vi "ReadMNValuesJSON_EditTolerance.vi"(7 "Default JSON\nVariant in":variant, 8 "error in":errorcluster, 9 "Part Name":string, 10 "Rack Number":string, 11 "JSON file path":path=path "C:/Users/raakeshs/Desktop/ppts/JSON/Write to JSON String/data/Files/test4.json") -> (0 "error out":errorcluster, 3 "Rack Controller Parameters":T1)   [LabVIEW 2015, in "ZenGage v3.0 UI.lvclass"]
uses:
  ZenGage v3.0 UI.lvclass
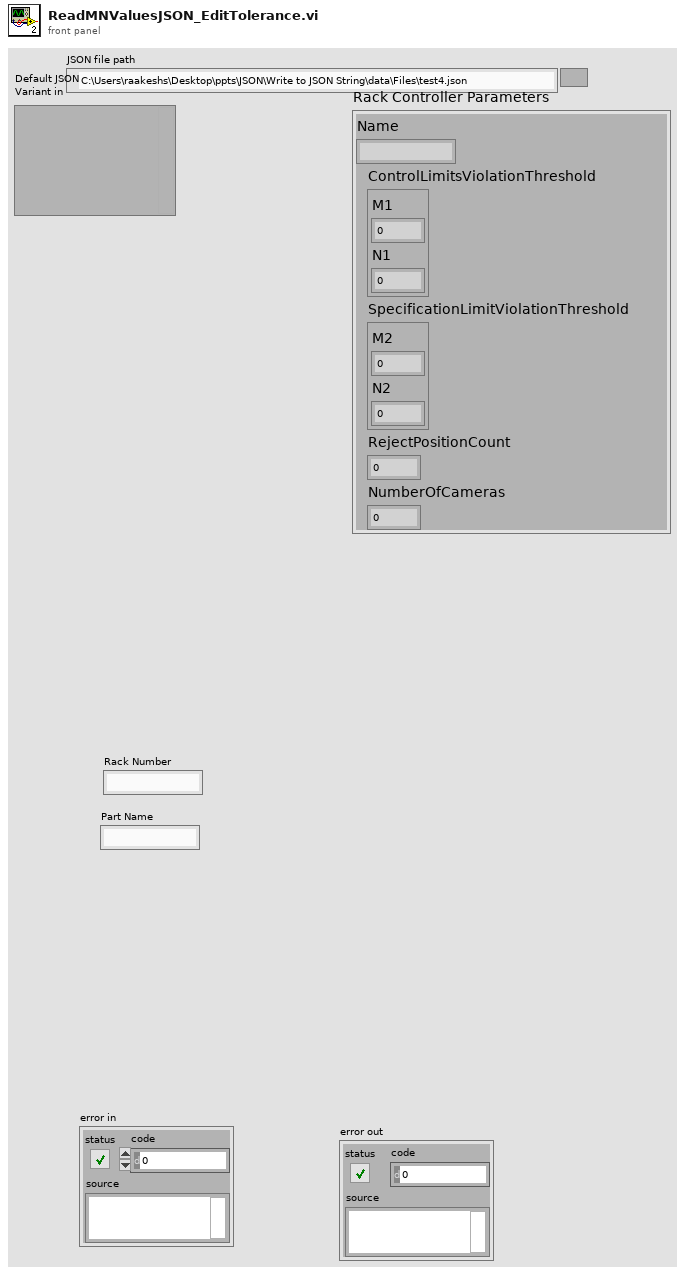
[diagram p1: front panel]
types:
  T1 = cluster{"Name":string, "ControlLimitsViolationThreshold":cluster{"M1":i32, "N1":i32}, "SpecificationLimitViolationThreshold":cluster{"M2":i32, "N2":i32}, "RejectPositionCount":i32, "NumberOfCameras":i32}
  T2 = cluster{cluster{"Name":string, "ControlLimitsViolationThreshold":cluster{"M1":i32, "N1":i32}, "SpecificationLimitViolationThreshold":cluster{"M2":i32, "N2":i32}, "RejectPositionCount":i32, "NumberOfCameras":i32}}
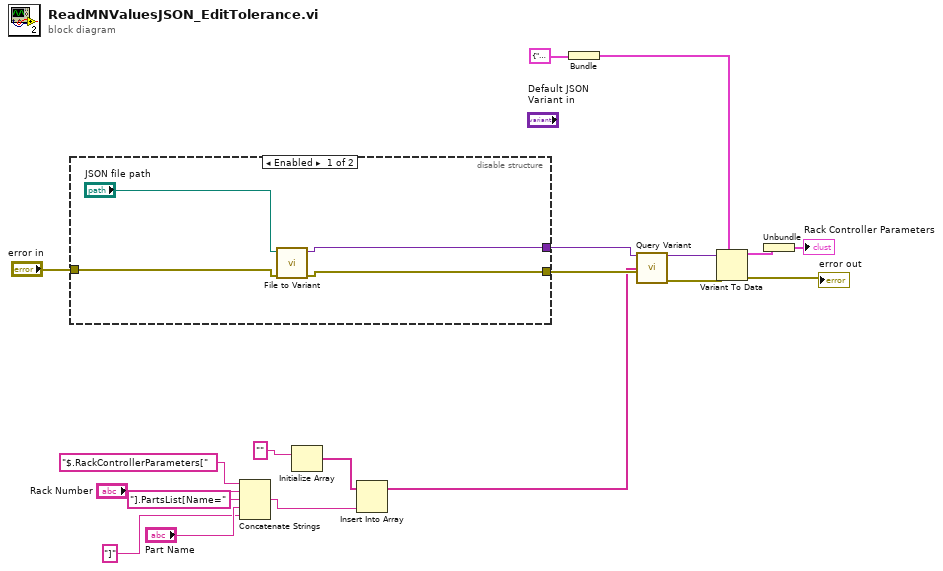
[diagram p0: block diagram]
diagram:
  n1 = disable-structure shown="Enabled" {
    disable-tunnel: [w22 w24] -> w19
    disable-tunnel: "error in" -> [w23 w24]
    disable-tunnel: [w20 _] -> w2
    frame Enabled {
      n2 = call <vilib>:"File to Variant.vi"("JSON FilePath"="JSON file path", "error in (no error)"=w23) -> ("JSON Variant"=w20:variant, "error out"=w22:errorcluster)  [unwired: 6 in, 1 out]
    }
    frame Disabled {
    }
  }
  n3 = Concatenate Strings("$.RackControllerParameters[" ("string"), "Rack Number", "].PartsList[Name=" ("string"), "Part Name", "]" ("string")) -> (w15:string)
  n4 = Initialize Array("") -> (w13:string[])  [unwired: 1 in]
  n5 = Insert Into Array(array=w13, new element=w15) -> (w12:string[])  [unwired: 1 in]
  n6 = Bundle(T1 {"Name"="", "ControlLimitsViolationThreshold"={"M1"=0, "N1"=0}, "SpecificationLimitViolationThreshold"={"M2"=0, "N2"=0}, "RejectPositionCount"=0, "NumberOfCameras"=0}) -> (w5:T2)  [unwired: 1 in]
  n7 = call <vilib>:"Query Variant.vi"("VCluster in"=w2, "pathList"=w12, "error IO"=w19) -> ("VCluster\n out"=w18:variant, "error out"=w16:errorcluster)  [unwired: 9 in, 2 out]
  n8 = Variant To Data(error in=w16, type=w5, Variant=w18) -> (data=w4:T2, error out=→"error out":errorcluster)
  n9 = Unbundle(w4) -> (→"Rack Controller Parameters":T1)
